vi "AgPSA _Launch Modular SA.vi"(7 "VISA resource name":refnum<visa-resource-name>="SpecAn_1", 8 "error in (no error)":errorcluster, 9 "Path":path=path "C:/Program Files/Agilent/SignalAnalysis/Infrastructure", 10 "Program":string="LaunchModularSA.exe PXI25::1::3::INSTR", 11 "Task Item":string="Agilent.SA.xSA.exe") -> (0 "error out":errorcluster, 3 "Success":bool=TRUE)   [LabVIEW 2015]
uses:
  <instrlib>/Agilent MXA Series/Agilent MXA Series.lvlib
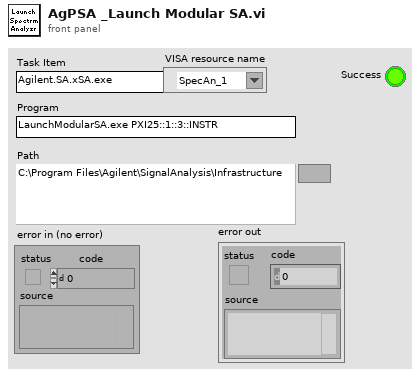
[diagram p1: front panel]
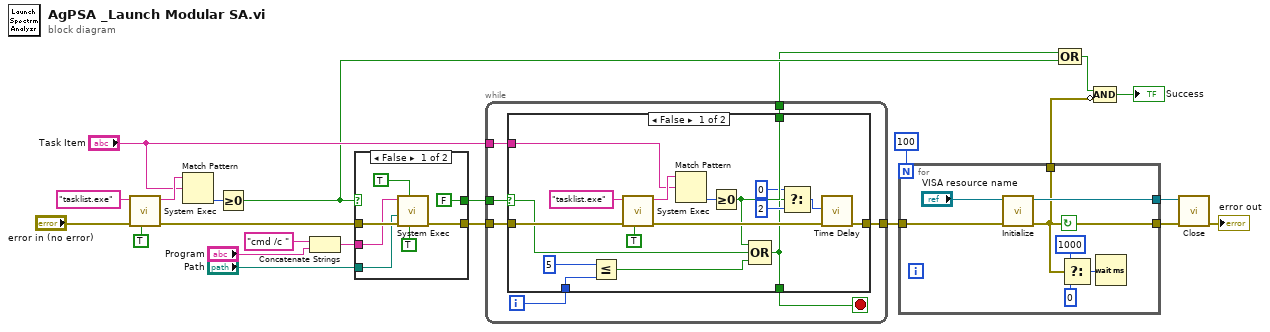
[diagram p0: block diagram]
diagram:
  n1 = call <vilib>:"System Exec.vi"("run minimized? (F)"=TRUE, "error in (no error)"="error in (no error)", "command line"="tasklist.exe") -> ("error out"=w19:errorcluster, "standard output"=w21:string)  [unwired: 5 in, 2 out]
  n2 = Match Pattern(string=w21, regular expression="Task Item") -> (offset past match=w20:i32)  [unwired: 1 in, 3 out]
  n3 = Greater Or Equal To 0?(x=w20) -> (x >= 0?=w14:bool)
  n4 = Concatenate Strings("cmd /c " ("command line"), "Program") -> (w10:string)
  n5 = case shown="False" w14 {
    selector: w14 -> [_ w32]
    tunnel: w19 -> [w30 w31]
    tunnel: "Path" -> [w29 _]
    tunnel: w10 -> [w28 _]
    tunnel: [w26 w31] -> w17
    tunnel: [FALSE w32] -> w16
    frame False {
      n6 = call <vilib>:"System Exec.vi"("run minimized? (F)"=TRUE, "wait until completion? (T)"=TRUE, "error in (no error)"=w30, "working directory"=w29, "command line"=w28) -> ("error out"=w26:errorcluster)  [unwired: 3 in, 3 out]
    }
    frame True {
    }
  }
  n7 = while {
    tunnel: w17 -> [w39]
    tunnel: w16 -> [w34]
    tunnel: "Task Item" -> [w38]
    tunnel: [w36] -> w13
    tunnel: [w33] -> w9
    i -> [w37]
    stop <- w35 stop-if-true
    n8 = case shown="False" w34 {
      selector: w34 -> [w41 w58]
      tunnel: w39 -> [w52 w57]
      tunnel: w38 -> [w51 _]
      tunnel: w37 -> [w50 _]
      tunnel: [w47 w58] -> w36
      tunnel: [w42 w58] -> w35
      tunnel: [w40 w57] -> w33
      frame False {
        n9 = Less Or Equal?(x=5, y=w50) -> (x <= y?=w43:bool)
        n10 = call <vilib>:"System Exec.vi"("run minimized? (F)"=TRUE, "error in (no error)"=w52, "command line"="tasklist.exe") -> ("error out"=w48:errorcluster, "standard output"=w55:string)  [unwired: 5 in, 2 out]
        n11 = Match Pattern(string=w55, regular expression=w51) -> (offset past match=w56:i32)  [unwired: 1 in, 3 out]
        n12 = Greater Or Equal To 0?(x=w56) -> (x >= 0?=w47:bool)
        n13 = Compound Arithmetic op=OR(w47, w41, w43) -> (w42:bool)
        n14 = Select(t=0 ("x"), s=w42, f=2 ("x")) -> (s? t:f=w44:i32)
        n15 = call "Time Delay"("error in (no error)"=w48, "Delay Time (s)"=w44) -> ("error out"=w40:errorcluster)  [unwired: 9 in]
      }
      frame True {
      }
    }
  }
  n16 = for {
    N: 100 ("x") -> [_]
    tunnel: w9 -> [w65]
    tunnel: [w63] -> w6
    tunnel: [w62] -> w5
    tunnel: [w62] -> w4
    stop <- w62 continue-if-true
    n17 = call <instrlib>:"Initialize.vi"("error in (no error)"=w65, "VISA resource name"="VISA resource name") -> ("error out"=w62:errorcluster, "VISA resource name out"=w63:refnum<visa-resource-name>)  [unwired: 8 in]
    n18 = Select(t=u32 1000 ("milliseconds to wait"), s=w62, f=u32 0) -> (s? t:f=w60:u32)
    n19 = Wait (ms)(milliseconds to wait=w60) -> ()  [unwired: 1 out]
  }
  n20 = Compound Arithmetic op=OR(w13, w14) -> (w8:bool)
  n21 = Compound Arithmetic op=AND(w8, invert w4) -> (→"Success":bool)
  n22 = call <instrlib>:"Close.vi"("error in (no error)"=w5, "VISA resource name"=w6) -> ("error out"=→"error out":errorcluster)  [unwired: 9 in]
